vi "JavaScript.vi"() -> ()   [LabVIEW 2017]
uses:
  <vilib>/Platform/browser.llb/Open URL in Default Browser (string).vi
  <vilib>/httpClient/POSTBuffer.vi
  <vilib>/httpClient/LabVIEWHTTPClient.lvlib
panel:
  out "body":string
  in  "dC":dbl(slide) scale=0.0..300.0
  in  "dB":dbl(slide) scale=0.0..300.0
  in  "dA":dbl(slide) scale=0.0..300.0
  in  "stop":bool
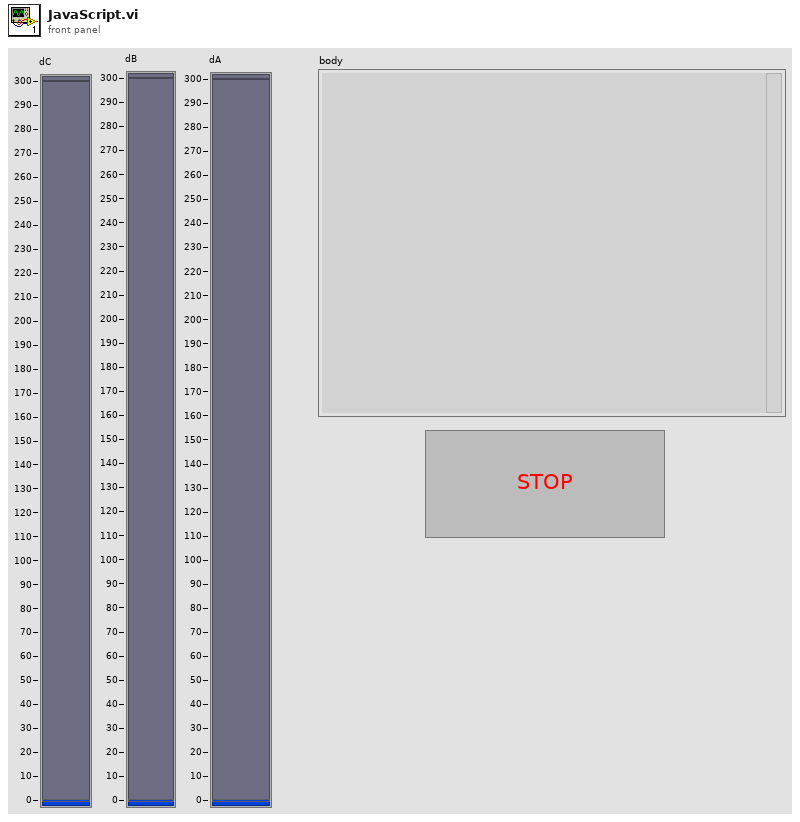
[diagram p1: front panel]
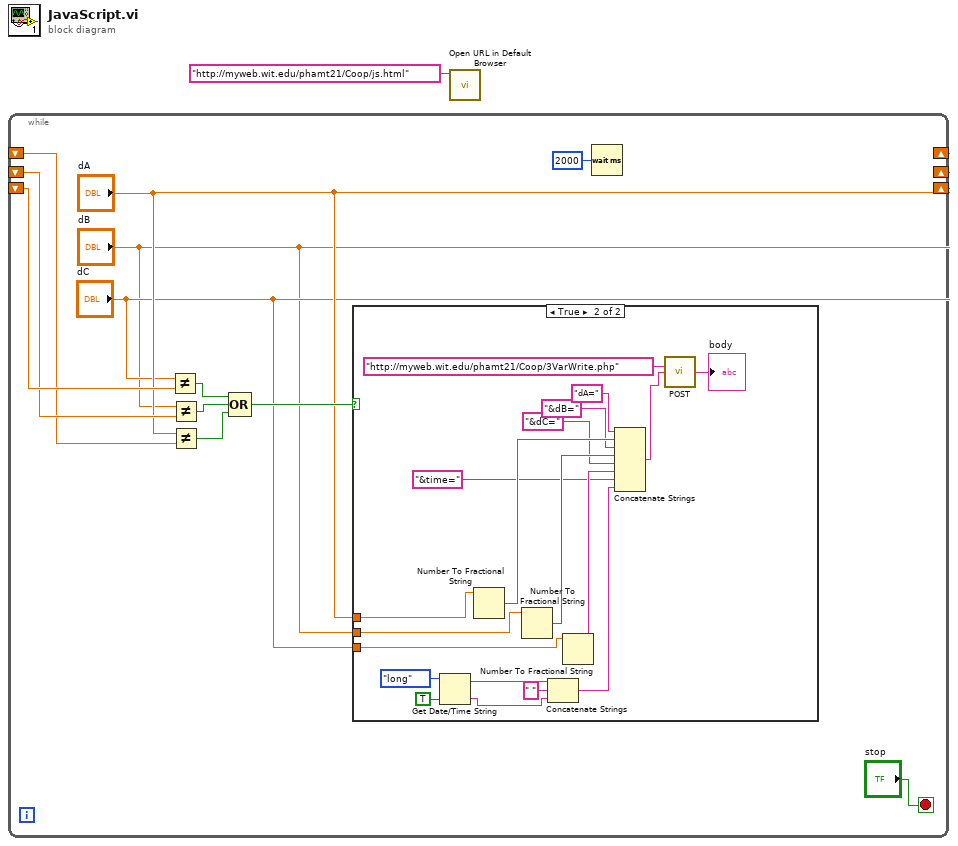
[diagram p0: block diagram]
diagram:
  n1 = while {
    shift-right: ["dC"] -> _
    shift-left: _ -> [w13]
    shift-right: ["dB"] -> _
    shift-left: _ -> [w8]
    shift-right: ["dA"] -> _
    shift-left: _ -> [w7]
    stop <- "stop" stop-if-true
    n2 = Not Equal?(x="dC", y=w13) -> (x != y?=w12:bool)
    n3 = Not Equal?(x="dB", y=w8) -> (x != y?=w11:bool)
    n4 = Not Equal?(x="dA", y=w7) -> (x != y?=w10:bool)
    n5 = Compound Arithmetic op=OR(w12, w11, w10) -> (w9:bool)
    n6 = case shown="True" w9 {
      tunnel: "dC" -> [_ w30]
      tunnel: "dB" -> [_ w31]
      tunnel: "dA" -> [_ w32]
      frame False {
      }
      frame True {
        n7 = Get Date/Time String(date format (0)=enum16{"short", "long", "abbreviated"}."long", want seconds? (F)=TRUE) -> (date string=w27:string, time string=w25:string)  [unwired: 1 in]
        n8 = Number To Fractional String(number=w32) -> (F-format string=w23:string)  [unwired: 3 in]
        n9 = Number To Fractional String(number=w31) -> (F-format string=w22:string)  [unwired: 3 in]
        n10 = Concatenate Strings(w27, " " ("string"), w25) -> (w20:string)
        n11 = Number To Fractional String(number=w30) -> (F-format string=w21:string)  [unwired: 3 in]
        n12 = Concatenate Strings("dA=" ("string"), w23, "&dB=" ("string"), w22, "&dC=" ("string"), w21, "&time=" ("string"), w20) -> (w19:string)
        n13 = call-poly <vilib>:"POST.vi"("url"="http://myweb.wit.edu/phamt21/Coop/3VarWrite.php", "buffer"=w19) -> ("body"=→"body":string)  [unwired: 10 in, 3 out]
      }
    }
    n14 = Wait (ms)(milliseconds to wait=u32 2000) -> ()  [unwired: 1 out]
  }
  n15 = call-poly <vilib>:"Open URL in Default Browser.vi"("URL"="http://myweb.wit.edu/phamt21/Coop/js.html") -> ()  [unwired: 5 in, 2 out]
